vi "DrawSite.vi"(4 "y corrector":dbl=1.0, 5 "Color":u32(colorbox)=16711680, 6 "x corrector":dbl=1.0, 7 "Group":string="Mask", 8 "error in (no error)":errorcluster, 9 "Position":cluster{"X":dbl, "Y":dbl, "Z":dbl, "Depth":dbl}, 10 "Scan Properties":T1={"X Size"=512.0, "Y Size"=512.0, "lens"=20.0, "mag"=1.0}, 11 "Image in":refnum<class "Image.lvclass">) -> (0 "error out":errorcluster, 3 "Image out":refnum<class "Image.lvclass">)   [LabVIEW 2012, in "Image.lvclass"]
uses:
  Image.lvclass
  Image.lvclass/Image.ctl
  <resource>/objmgr/IMAQImage.rc
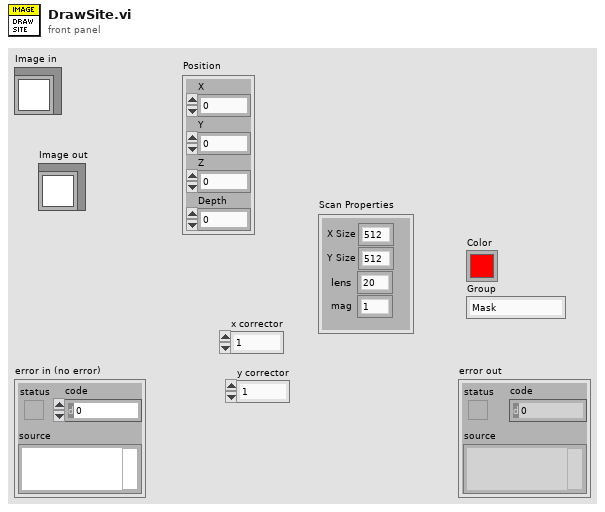
[diagram p1: front panel]
types:
  T1 = cluster{"X Size":dbl, "Y Size":dbl, "lens":dbl, "mag":dbl}
  T2 = cluster{"Left":i32, "Top":i32, "Right":i32, "Bottom":i32}
  T3 = typedef "IMAQ Image.ctl" = refnum<image>
  T4 = cluster{"scan_idx":i32, "lens":i32, "mag":dbl, "x":dbl, "y":dbl, "mouse_id":i32, "exp_date":string, "file_name":string, "file_path":path}
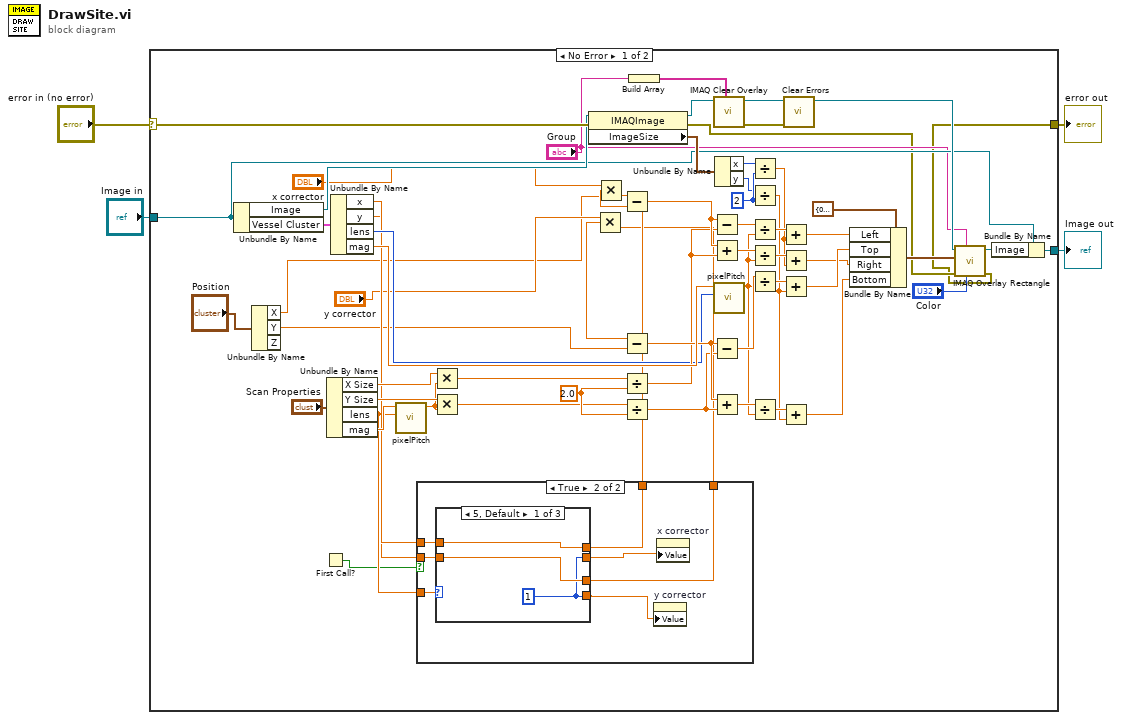
[diagram p0: block diagram]
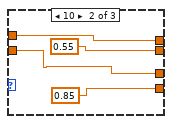
[diagram p3: hidden frame]
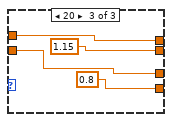
[diagram p4: hidden frame]
diagram:
  n1 = case shown="No Error" "error in (no error)" {
    selector: "error in (no error)" -> [w25 w88]
    tunnel: [w17 w88] -> w3
    tunnel: [w21 w87] -> w1
    tunnel: "Image in" -> [w22 w87]
    frame No Error {
      w50 = 2.0 ("y")
      w65 = 2 ("y")
      n2 = Unbundle By Name(w22) -> ("Image"=w24:T3, "Vessel Cluster"=w23:T4)
      n3 = Unbundle By Name("Position") -> ("X"=w6:dbl, "Y"=w5:dbl)  [unwired: 1 out]
      n4 = First Call?() -> (First Call?: T/F=w9:bool)
      n5 = Unbundle By Name("Scan Properties") -> ("X Size"=w49:dbl, "Y Size"=w48:dbl, "lens"=w26:dbl, "mag"=w57:dbl)
      n6 = Unbundle By Name(w23) -> ("x"=w28:dbl, "y"=w27:dbl, "lens"=w29:i32, "mag"=w58:dbl)
      n7 = call "pixelPitch.vi"("Lens"=w26, "Mag"=w57) -> ("PixelPitch"=w47:dbl)  [unwired: 9 in]
      n8 = case shown="True" w9 {
        tunnel: w28 -> [w68 w75]
        tunnel: w27 -> [w67 w74]
        tunnel: w26 -> [_ w73]
        tunnel: [w68 w72] -> w15
        tunnel: [w67 w71] -> w11
        frame False {
        }
        frame True {
          n9 = case shown="5, Default" w73 {
            tunnel: w75 -> [w78 w82 w86]
            tunnel: [w78 w82 w86] -> w72
            tunnel: w74 -> [w77 w80 w85]
            tunnel: [w77 w80 w85] -> w71
            tunnel: [w76 0.55 ("x") 1.15] -> w70
            tunnel: [w76 0.85 ("y") 0.8] -> w69
            frame 5, Default {
              w76 = 1
            }
            frame 10 {
            }
            frame 20 {
            }
          }
          n10 = property on="y corrector" class="DigNum (strict)"("Value"=w69) -> ()  [unwired: 2 in, 2 out]
          n11 = property on="x corrector" class="DigNum (strict)"("Value"=w70) -> ()  [unwired: 2 in, 2 out]
        }
      }
      n12 = Multiply(x=w49, y=w47) -> (x*y=w45:dbl)
      n13 = Multiply(x=w48, y=w47) -> (x*y=w44:dbl)
      n14 = property class="IMAQImage"(reference=w24, error in=w25) -> (reference out=w60:T3, error out=w18:errorcluster, "ImageSize"=w63:cluster{"x":i32, "y":i32})
      n15 = Multiply(x="y corrector", y=w11) -> (x*y=w12:dbl)
      n16 = Multiply(x="x corrector", y=w15) -> (x*y=w14:dbl)
      n17 = Subtract(x=w6, y=w14) -> (x-y=w32:dbl)
      n18 = Subtract(x=w12, y=w5) -> (x-y=w33:dbl)
      n19 = Divide(x=w45, y=w50) -> (x/y=w31:dbl)
      n20 = Divide(x=w44, y=w50) -> (x/y=w30:dbl)
      n21 = Build Array("Group") -> (w19:string[])
      n22 = Subtract(x=w32, y=w31) -> (x-y=w51:dbl)
      n23 = Add(x=w32, y=w31) -> (x+y=w54:dbl)
      n24 = Subtract(x=w33, y=w30) -> (x-y=w52:dbl)
      n25 = Add(x=w33, y=w30) -> (x+y=w53:dbl)
      n26 = call "IMAQ Clear Overlay"("Groups"=w19, "Image"=w60) -> ("error out"=w16:errorcluster, "Image Out"=w64:T3)  [unwired: 1 in, 7 out]
      n27 = call "pixelPitch.vi"("Lens"=w29, "Mag"=w58) -> ("PixelPitch"=w46:dbl)  [unwired: 9 in]
      n28 = Unbundle By Name(w63) -> ("x"=w62:i32, "y"=w61:i32)
      n29 = Divide(x=w62, y=w65) -> (x/y=w35:dbl)
      n30 = Divide(x=w61, y=w65) -> (x/y=w34:dbl)
      n31 = Divide(x=w51, y=w46) -> (x/y=w43:dbl)
      n32 = Divide(x=w54, y=w46) -> (x/y=w41:dbl)
      n33 = Divide(x=w52, y=w46) -> (x/y=w42:dbl)
      n34 = Divide(x=w53, y=w46) -> (x/y=w40:dbl)
      n35 = Add(x=w43, y=w35) -> (x+y=w39:dbl)
      n36 = Add(x=w41, y=w35) -> (x+y=w37:dbl)
      n37 = Add(x=w42, y=w34) -> (x+y=w38:dbl)
      n38 = Add(x=w40, y=w34) -> (x+y=w36:dbl)
      n39 = call <vilib>:"Clear Errors.vi"("error in (no error)"=w16) -> ()  [unwired: 6 in, 1 out]
      n40 = Bundle By Name(cluster=T2 {"Left"=0, "Top"=0, "Right"=0, "Bottom"=0} ("Rectangle"), "Left"=w39, "Top"=w38, "Right"=w37, "Bottom"=w36) -> (w55:T2)
      n41 = call "IMAQ Overlay Rectangle"("Color"="Color", "Group"="Group", "error in (no error)"=w18, "Rectangle"=w55, "Image"=w64) -> ("error out"=w17:errorcluster, "Image Out"=w8:T3)  [unwired: 5 in]
      n42 = Bundle By Name(cluster=w22, "Image"=w8) -> (w21:refnum<class "Image.lvclass">)
    }
    frame Error {
    }
  }
  "error out" <- w3
  "Image out" <- w1
